vi "Create Channel.vi"(6 "RDB Signalname":string, 7 "PlayerID":u8=1, 8 "error in (no error)":errorcluster, 9 "Channel":T2, 10 "RDB Receive Objects":string, 11 "Item Ref in":T1 format="%.0x") -> (0 "error out":errorcluster)   [LabVIEW 2023, in "Vires VTD System Explorer.lvlib"]
uses:
  Vires VTD System Explorer.lvlib
  <vilib>/NI VeriStand/Custom Device API/Custom Device Channel.ctl
  <vilib>/NI VeriStand/Custom Device API/Custom Device Channel Type.ctl
  <vilib>/NI VeriStand/Custom Device API/Custom Device Item Ref.ctl
  <vilib>/xnet/xnet.llb/XNET String To IO Name (Signal).vi
  Shared/Constants.vi
  <vilib>/NI VeriStand/Custom Device API/Custom Device API.lvlib
  Shared/Vires VTD Shared.lvlib
  <resource>/objmgr/xnet.rc
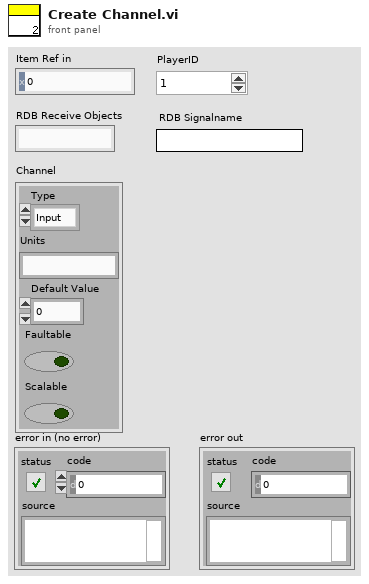
[diagram p1: front panel]
types:
  T1 = typedef "Custom Device API.lvlib/Custom Device Item Ref.ctl" = u64
  T2 = typedef "Custom Device API.lvlib/Custom Device Channel.ctl" = cluster{"Type":T3, "Units":string, "Default Value":dbl, "Faultable":bool, "Scalable":bool}
  T3 = typedef "Custom Device API.lvlib/Custom Device Channel Type.ctl" = enum16{"Input", "Output"}
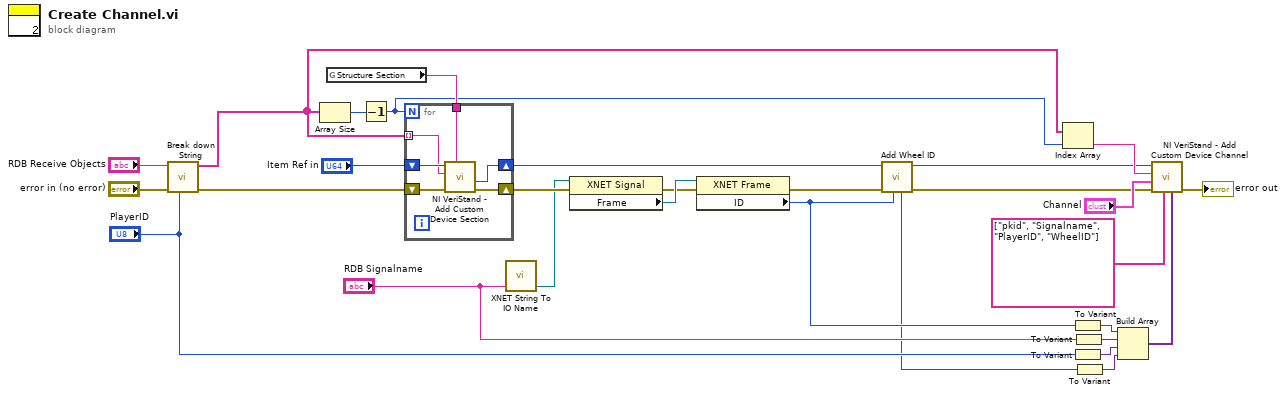
[diagram p0: block diagram]
diagram:
  n1 = call "Break down String.vi"("PlayerID"="PlayerID", "Error in"="error in (no error)", "Input String"="RDB Receive Objects") -> ("Error Out"=w24:errorcluster, "Output"=w22:string[])  [unwired: 7 in]
  n2 = Array Size(array=w22) -> (size(s)=w23:i32)
  n3 = global read "Constants.vi" "Structure Section"() -> (w26:string)
  n4 = Decrement(x=w23) -> (x-1=w21:i32)
  n5 = for {
    N: w21 -> [_]
    tunnel: w26 -> [w34]
    shift-right: [w30] -> w5
    shift-left: "Item Ref in" -> [w35]
    shift-right: [w32] -> w11
    shift-left: w24 -> [w33]
    tunnel: w22 -> [w31] mode=indexing
    n6 = call <vilib>:"NI VeriStand - Add Custom Device Section.vi"("GUID (Default Section)"=w34, "error in (no error)"=w33, "Section Name"=w31, "Parent Ref in"=w35) -> ("error out"=w32:errorcluster, "Section Ptr"=w30:T1)  [unwired: 4 in, 2 out]
  }
  n7 = call-poly <vilib>:"XNET String To IO Name.vi"("string"="RDB Signalname") -> ("XNET Signal"=w10:refnum<k21>)  [unwired: 4 out]
  n8 = property class="XNET Signal"(reference=w10, error in=w11) -> (error out=w12:errorcluster, "Frame"=w13:refnum<k21>)  [unwired: 1 out]
  n9 = property class="XNET Frame"(reference=w13, error in=w12) -> (error out=w7:errorcluster, "ID"=w3:u32)  [unwired: 1 out]
  n10 = call "Add Wheel ID.vi"("Identifier"=w3, "error in (no error)"=w7, "Item Ref in"=w5) -> ("error out"=w6:errorcluster, "Item Ref out"=w4:T1, "WheelID"=w1:i32)  [unwired: 6 in]
  n11 = Index Array(array=w22, index=w21) -> (element=w20:string)
  n12 = To Variant(anything=w3) -> (Variant=w8:variant)
  n13 = To Variant(anything="PlayerID") -> (Variant=w15:variant)
  n14 = To Variant(anything="RDB Signalname") -> (Variant=w18:variant)
  n15 = To Variant(anything=w1) -> (Variant=w2:variant)
  n16 = Build Array(w8, w18, w15, w2) -> (w17:variant[])
  n17 = call <vilib>:"NI VeriStand - Add Custom Device Channel.vi"("Property Values"=w17, "Property names"=string[] ["pkid", "Signalname", "PlayerID", "WheelID"], "error in (no error)"=w6, "Channel"="Channel", "Channel Name"=w20, "Parent Ref in"=w4) -> ("error out"=→"error out":errorcluster)  [unwired: 2 in, 3 out]
